vi "Update Boolean Value.vi"(9 "Value":bool, 10 "Tree Tag":string, 11 "UI Data in":refnum<class "Settings UI.lvclass">) -> (3 "UI Data out":refnum<class "Settings UI.lvclass">)   [LabVIEW 2024, in "Output Sequencer.lvlib" / "Settings UI.lvclass"]
uses:
  Settings UI.lvclass
  Settings UI.lvclass/Settings UI.ctl
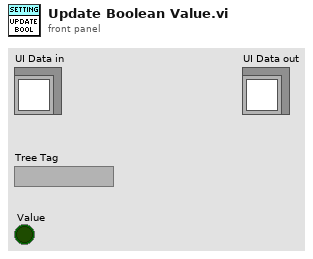
[diagram p1: front panel]
types:
  T1 = typedef "Output Sequencer.lvlib/Settings UI.lvclass/Tree Index Enum.ctl" = enum16{"General Settings", "Num Steps", "Num Analog", "Num Digital", "Show Confirmation", "Interp Priority", "Adv Timing", "Enable Conditions", "Seq Execution", "Reset Test Start", "Only When Test", "Delay After Test", "Start condition", "Re-triggering", "Stop condition", "Stop After Cycles", "Stop Values", "Default Values", "Default Analog", "Default Digital", "Steps", "Step #", "Description", "Precondition", "Duration", "Mode", "Delay Between Vals", "Analog Values", "Digital Values", "Postcondition", "On True", "On False"}
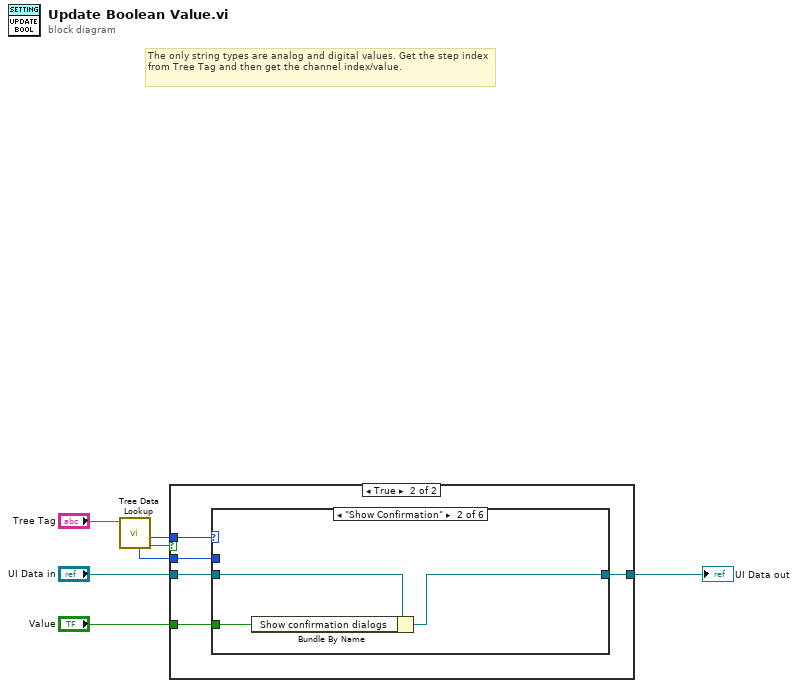
[diagram p0: block diagram]
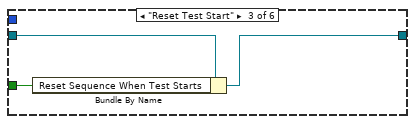
[diagram p4: hidden frame]
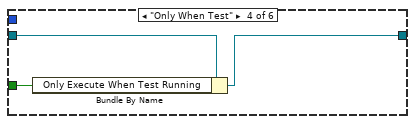
[diagram p5: hidden frame]
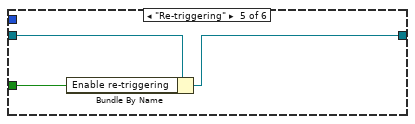
[diagram p6: hidden frame]
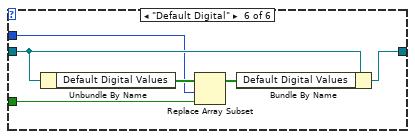
[diagram p7: hidden frame]
diagram:
  # "The only string types are analog and digital values. Get the step index from Tree Tag and then get the channel index/value."
  n1 = call "Tree Data Lookup.vi"("Tag in"="Tree Tag") -> ("Found?"=w3:bool, "Tree Index Enum"=w2:T1, "Item Number"=w1:i32)  [unwired: 5 in, 3 out]
  n2 = case shown="True" w3 {
    tunnel: "UI Data in" -> [w8 w13]
    tunnel: "Value" -> [_ w12]
    tunnel: [w8 w11] -> w4
    tunnel: w2 -> [_ w10]
    tunnel: w1 -> [_ w9]
    frame False {
    }
    frame True {
      n3 = case shown="\"Show Confirmation\"" w10 {
        tunnel: w13 -> [w14 w16 w20 w23 w26 w29]
        tunnel: w12 -> [_ w17 w19 w22 w25 w27]
        tunnel: [w14 w15 w18 w21 w24 w30] -> w11
        tunnel: w9 -> [_ _ _ _ _ w28]
        frame Default {
        }
        frame "Show Confirmation" {
          n4 = Bundle By Name(cluster=w16, "Show confirmation dialogs"=w17) -> (w15:refnum<class "Settings UI.lvclass">)
        }
        frame "Reset Test Start" {
          n5 = Bundle By Name(cluster=w20, "Reset Sequence When Test Starts"=w19) -> (w18:refnum<class "Settings UI.lvclass">)
        }
        frame "Only When Test" {
          n6 = Bundle By Name(cluster=w23, "Only Execute When Test Running"=w22) -> (w21:refnum<class "Settings UI.lvclass">)
        }
        frame "Re-triggering" {
          n7 = Bundle By Name(cluster=w26, "Enable re-triggering"=w25) -> (w24:refnum<class "Settings UI.lvclass">)
        }
        frame "Default Digital" {
          n8 = Unbundle By Name(w29) -> ("Default Digital Values"=w32:bool[])
          n9 = Replace Array Subset(array=w32, new element=w27, index=w28) -> (w31:bool[])
          n10 = Bundle By Name(cluster=w29, "Default Digital Values"=w31) -> (w30:refnum<class "Settings UI.lvclass">)
        }
      }
    }
  }
  "UI Data out" <- w4
